vi "solar_read MainQ.vi"(8 "error in (no error)":errorcluster, 11 "solar in":refnum<class "solar.lvclass">) -> (0 "error out":errorcluster, 2 "Queue":refnum<queue>, 3 "solar out":refnum<class "solar.lvclass">)   [LabVIEW 2018, in "solar.lvclass"]
doc: "This returns the top level main target queue reference."
uses:
  solar.lvclass
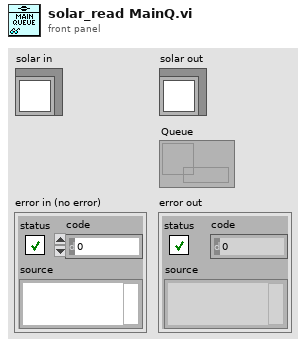
[diagram p1: front panel]
types:
  T1 = typedef "solar_ctl SOLAR Refnum.ctl" = refnum<k1>
  T2 = typedef "solar_ctl SOLAR Global.ctl" = cluster{"Targets":T3[], "AppDir":path, "solar.ini":path, "ConfigsDir":path, "CosmosDir":path, "LogsDir":path, "ExePath":path, "ExeVersion":string, "PartNum":string, "AppSetup":string, "Title":string, "Main.ini":path, "Temp.ini":path, "vSOLAR":string, "Splash.png":string, "SplashWait":i32, "SOLARUE":refnum<user-event>, "VoyagerRefnum":T4, "QTimerRefnum":T5}
  T3 = typedef "solar_ctl Target Global.ctl" = cluster{"Target":string, "Q":refnum<queue>, "UE":refnum<user-event>, "VI":refnum<vi>, "Menu":refnum<k9>, "Data":refnum<data-value>, "Attributes":variant}
  T4 = typedef "solar_voy_ctl Voyager Refnum.ctl" = refnum<k1>
  T5 = typedef "solar_qtimer_ctl Refnum.ctl" = refnum<k1>
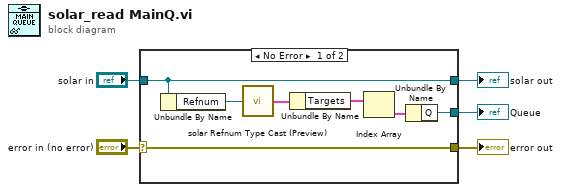
[diagram p0: block diagram]
diagram:
  n1 = case shown="No Error" "error in (no error)" {
    selector: "error in (no error)" -> [w7 w14]
    tunnel: "solar in" -> [w6 w13]
    tunnel: [w8 _] -> w1
    tunnel: [w7 w14] -> w4
    tunnel: [w6 w13] -> w2
    frame No Error {
      n2 = Unbundle By Name(w6) -> ("Refnum"=w12:T1)
      n3 = call "solar Refnum Type Cast (Preview).vi"("Refnum"=w12) -> ("SOLAR"=w11:T2)  [unwired: 8 in]
      n4 = Unbundle By Name(w11) -> ("Targets"=w10:T3[])
      n5 = Index Array(array=w10) -> (element=w9:T3)  [unwired: 1 in]
      n6 = Unbundle By Name(w9) -> ("Q"=w8:refnum<queue>)
    }
    frame Error {
    }
  }
  "error out" <- w4
  "solar out" <- w2
  "Queue" <- w1
